vi "write_log_metadata.vi"(8 "error in (no error)":errorcluster, 10 "data":variant, 11 "lfield_logger in":refnum<class "lfield_logger.lvclass">) -> (0 "error out":errorcluster, 3 "lfield_logger out":refnum<class "lfield_logger.lvclass">)   [LabVIEW 2015, in "lfield_logger.lvclass"]
uses:
  lfield_logger.lvclass
  metadata_tdef.ctl
  lfield_logger.lvclass/lfield_logger.ctl
  <vilib>/UPVI/lvhdf5/attribute.llb/LVH5A Operation.ctl
  <vilib>/UPVI/lvhdf5/attribute.llb/Simple H5Awrite (Variant).vi
  <vilib>/UPVI/lvhdf5/attribute.llb/Simple H5Awrite.xnode
  <vilib>/UPVI/lvhdf5/library.llb/HDF5 Ref.ctl
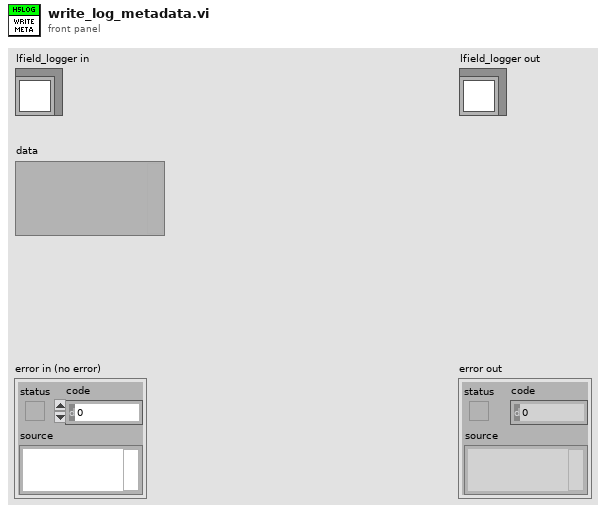
[diagram p1: front panel]
types:
  T1 = typedef "metadata_tdef.ctl" = cluster{"notes":string}
  T2 = typedef "LVH5A Operation.ctl" = enum16{"open", "replace", "create", "open or create", "create or replace", "create or replace with confirmation"}
  T3 = typedef "HDF5 Ref.ctl" = refnum<k1>
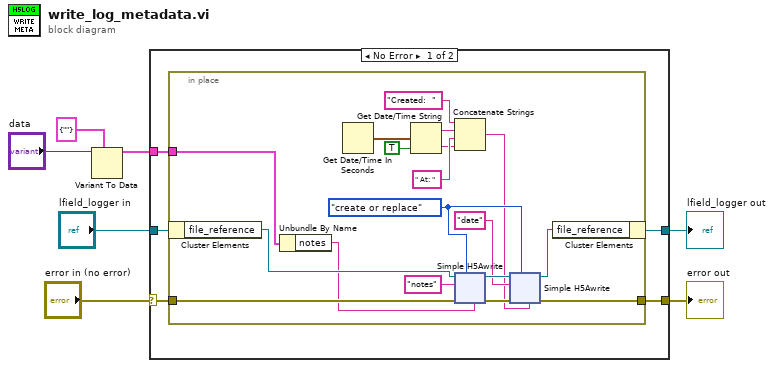
[diagram p0: block diagram]
diagram:
  n1 = Variant To Data(type=T1 {"notes"=""} ("output cluster"), Variant="data") -> (data=w3:T1)  [unwired: 1 in, 1 out]
  n2 = case shown="No Error" "error in (no error)" {
    selector: "error in (no error)" -> [w11 w61]
    tunnel: "lfield_logger in" -> [w12 w62]
    tunnel: w3 -> [w10 _]
    tunnel: [w9 w61] -> w2
    tunnel: [w8 w62] -> w1
    frame No Error {
      n3 = in-place {
        in-place-border: w11 -> [w28]
        in-place-border: w10 -> [w27]
        in-place-border: [w13] -> w9
        w16 = LVH5A_Operation."create or replace" ("operation (open or create)")
        n4 = in-place-cluster #1(w12) -> ("file_reference"=w30:T3)
        n5 = Unbundle By Name(w27) -> ("notes"=w26:string)
        n6 = Get Date/Time In Seconds() -> (seconds since 1Jan1904=w25:timestamp)
        n7 = Get Date/Time String(seconds (now)=w25, want seconds? (F)=TRUE) -> (date string=w23:string, time string=w21:string)  [unwired: 1 in]
        n8 = Concatenate Strings("Created:  " ("string"), w23, " At: " ("string"), w21) -> (w15:string)
        n9 = xnode "Simple H5Awrite"("HDF5 Ref"=w30, "Name"="notes", "error in (no error)"=w28, "operation (open or create)"=w16, "Value"=w26) -> ("HDF5 Ref out"=w18:T3, "error out"=w19:errorcluster)
        n10 = xnode "Simple H5Awrite"("HDF5 Ref"=w18, "Name"="date", "error in (no error)"=w19, "operation (open or create)"=w16, "Value"=w15) -> ("HDF5 Ref out"=w14:T3, "error out"=w13:errorcluster)
        n11 = in-place-cluster #1("file_reference"=w14) -> (w8:refnum<class "lfield_logger.lvclass">)
      }
    }
    frame Error {
    }
  }
  "error out" <- w2
  "lfield_logger out" <- w1
